vi "VI Tree.vi"   [LabVIEW 2018, in "Agilent U2722.lvlib"]
doc: "This is the instrument driver for the Agilent U2722A and U2723A USB Modular Source Measure Unit. The VI Tree displays all the user-callable VIs of the instrument driver in an organized table."
uses:
  <instrlib>/Agilent U2722/Agilent U2722.lvlib
  <instrlib>/Agilent U2722/Public/Configure/Configure Channel (Current).vi
  <instrlib>/Agilent U2722/Public/Data/Read Output (Single).vi
panel:
  # "(c) 2009-2015 National Instruments.  ALL RIGHTS RESERVED."
  # "SEE DIAGRAM\nFOR VI TREE."
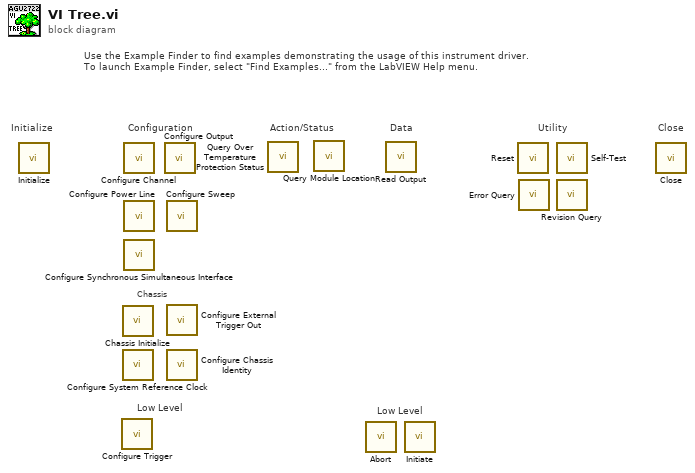
[diagram p0: block diagram]
diagram:
  # "Low Level"
  # "Chassis"
  # "Low Level"
  # "Use the Example Finder to find examples demonstrating the usage of this instrument driver.\nTo launch Example Finder, select \"Find Examples...\" from the LabVIEW Help menu."
  # "Configuration"
  # "Utility"
  # "Data"
  # "Action/Status"
  # "Close"
  # "Initialize"
  n1 = call <instrlib>:"Initialize.vi"() -> ()  [unwired: 10 in, 2 out]
  n2 = call <instrlib>:"Configure Trigger.vi"() -> ()  [unwired: 10 in, 2 out]
  n3 = call <instrlib>:"Chassis Initialize.vi"() -> ()  [unwired: 10 in, 2 out]
  n4 = call <instrlib>:"Configure System Reference Clock.vi"() -> ()  [unwired: 10 in, 2 out]
  n5 = call-poly <instrlib>:"Configure Channel.vi"() -> ()  [unwired: 10 in, 2 out]
  n6 = call <instrlib>:"Configure Power Line.vi"() -> ()  [unwired: 10 in, 2 out]
  n7 = call <instrlib>:"Configure Synchronous Simultaneous Interface.vi"() -> ()  [unwired: 10 in, 2 out]
  n8 = call <instrlib>:"Configure Output.vi"() -> ()  [unwired: 10 in, 2 out]
  n9 = call <instrlib>:"Configure Sweep.vi"() -> ()  [unwired: 10 in, 2 out]
  n10 = call <instrlib>:"Configure External Trigger Out.vi"() -> ()  [unwired: 10 in, 2 out]
  n11 = call <instrlib>:"Configure Chassis Identity.vi"() -> ()  [unwired: 10 in, 2 out]
  n12 = call <instrlib>:"Query Over Temperature Protection Status.vi"() -> ()  [unwired: 9 in, 3 out]
  n13 = call <instrlib>:"Query Module Location.vi"() -> ()  [unwired: 8 in, 4 out]
  n14 = call <instrlib>:"Abort.vi"() -> ()  [unwired: 10 in, 2 out]
  n15 = call-poly <instrlib>:"Read Output.vi"() -> ()  [unwired: 8 in, 4 out]
  n16 = call <instrlib>:"Initiate.vi"() -> ()  [unwired: 10 in, 2 out]
  n17 = call <instrlib>:"Reset.vi"() -> ()  [unwired: 10 in, 2 out]
  n18 = call <instrlib>:"Error Query.vi"() -> ()  [unwired: 8 in, 4 out]
  n19 = call <instrlib>:"Self-Test.vi"() -> ()  [unwired: 8 in, 4 out]
  n20 = call <instrlib>:"Revision Query.vi"() -> ()  [unwired: 8 in, 4 out]
  n21 = call <instrlib>:"Close.vi"() -> ()  [unwired: 11 in, 1 out]
